vi "Keyence LJ-V7000 Read Batch Profiles(for High-Speed Mode).vi"() -> ()   [LabVIEW 2014]
doc: "This example mainly indicates how to acquire profiles in a unit of batch from controllers by using <B>Read Batch Profiles (for High-Speed Mode)</B> VI. \n\n<B>Note</B>:\nIf you execute this example, set the operation mode of the controller to the high-speed mode, and set batch measurement to ON in batch setting."
uses:
  Public/constant/Comm Interface.ctl
  Public/Clusters/Ethernet Config.ctl
  Public/Clusters/Read Batch Profile Req.ctl
  Public/constant/Batch Pos.ctl
  Public/Clusters/Read Batch Profile Rsp.ctl
  Public/Clusters/Profile Info.ctl
  State Machine State1.ctl
  Keyence LJ-V7000.lvlib
panel:
  in  "Start Monitoring":bool
  in  "Batch Stop":bool
  in  "Batch Start":bool
  out "Batch Height Image":dbl[][](graph)
  out "Profile Info":T1
  out "Profile Rsp":T2
  in  "Batch Point":u16=1000
  in  "Read Req":T3={"Read Area"=TRUE, "Batch Pos"=0, "Read Batch No"=0, "Read Profile No."=0, "Read Profile Cnt"=255, "Erase"=FALSE} {"Batch Pos" items=["CURRENT"=0, "SPECIFY"=2, "COMMITED"=3, "NEWEST PROFILE"=4]}
  in  "Stop VI":bool
  in  "Ethernet Config":T5={"IP Address"=[192, 168, 0, 1], "Port No"=24691}
  in  "Comm Interface":T6
  # "Communication Configuration"
  # "Output from Read Profiles VI"
  # "Input to Read Profiles VI"
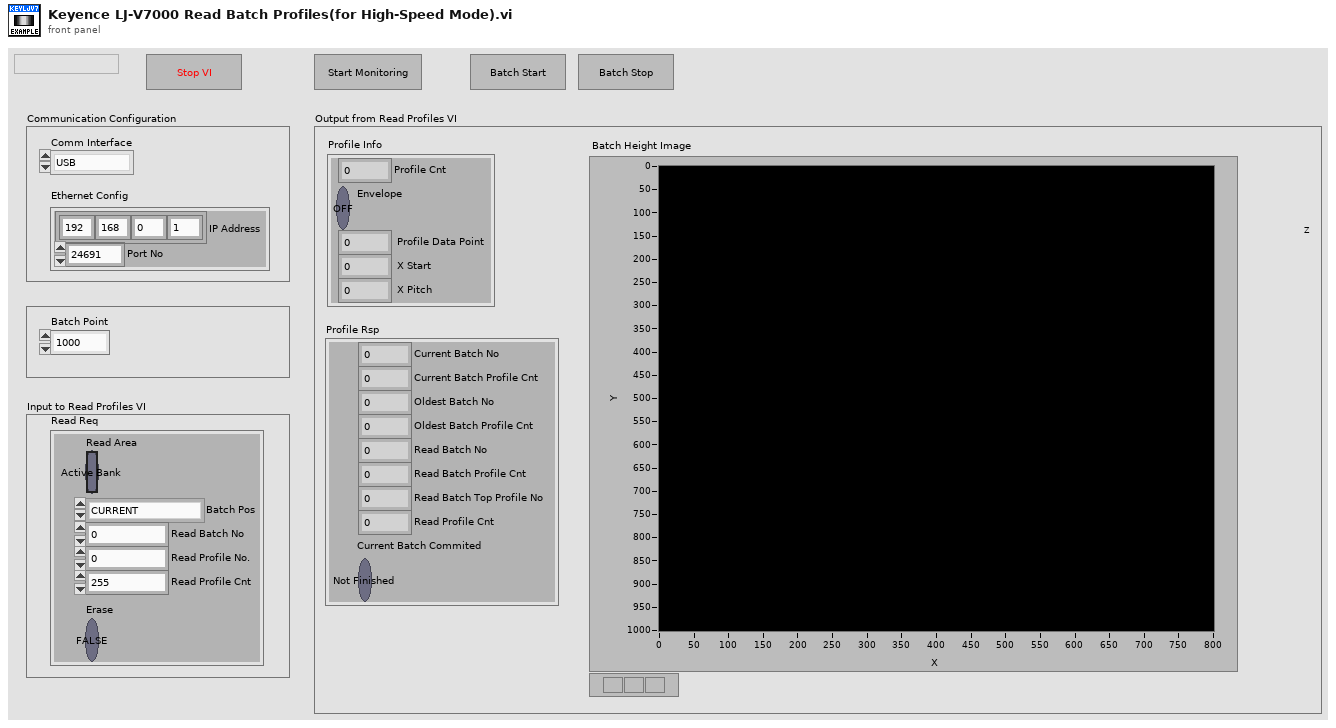
[diagram p1: front panel]
types:
  T1 = typedef "Keyence LJ-V7000.lvlib/Profile Info.ctl" = cluster{"Profile Cnt":u8, "Envelope":bool, " Profile Data Point":u16, " X Start":i32, " X Pitch":i32}
  T2 = typedef "Keyence LJ-V7000.lvlib/Read Batch Profile Rsp.ctl" = cluster{"Current Batch No":u32, "Current Batch Profile Cnt":u32, "Oldest Batch No":u32, "Oldest Batch Profile Cnt":u32, "Read Batch No":u32, "Read Batch Profile Cnt":u32, "Read Batch Top Profile No":u32, "Read Profile Cnt":u8, "Current Batch Commited":bool}
  T3 = typedef "Keyence LJ-V7000.lvlib/Read Batch Profile Req.ctl" = cluster{"Read Area":bool, "Batch Pos":T4, "Read Batch No":u32, "Read Profile No.":u32, "Read Profile Cnt":u8, "Erase":bool}
  T4 = typedef "Keyence LJ-V7000.lvlib/Batch Pos.ctl" = u8
  T5 = typedef "Keyence LJ-V7000.lvlib/Ethernet Config.ctl" = cluster{"IP Address":u8[], "Port No":u16}
  T6 = typedef "Keyence LJ-V7000.lvlib/Comm Interface.ctl" = enum8{"USB", "ETHERNET"}
  T7 = typedef "State Machine State1.ctl" = enum16{"Idle", "Batch Reading Initialize", "Batch Reading", "Batch Start", "Batch Stop", "Stop"}
  T8 = enum8{"Enabled", "Disabled", "Disabled and Grayed Out"}
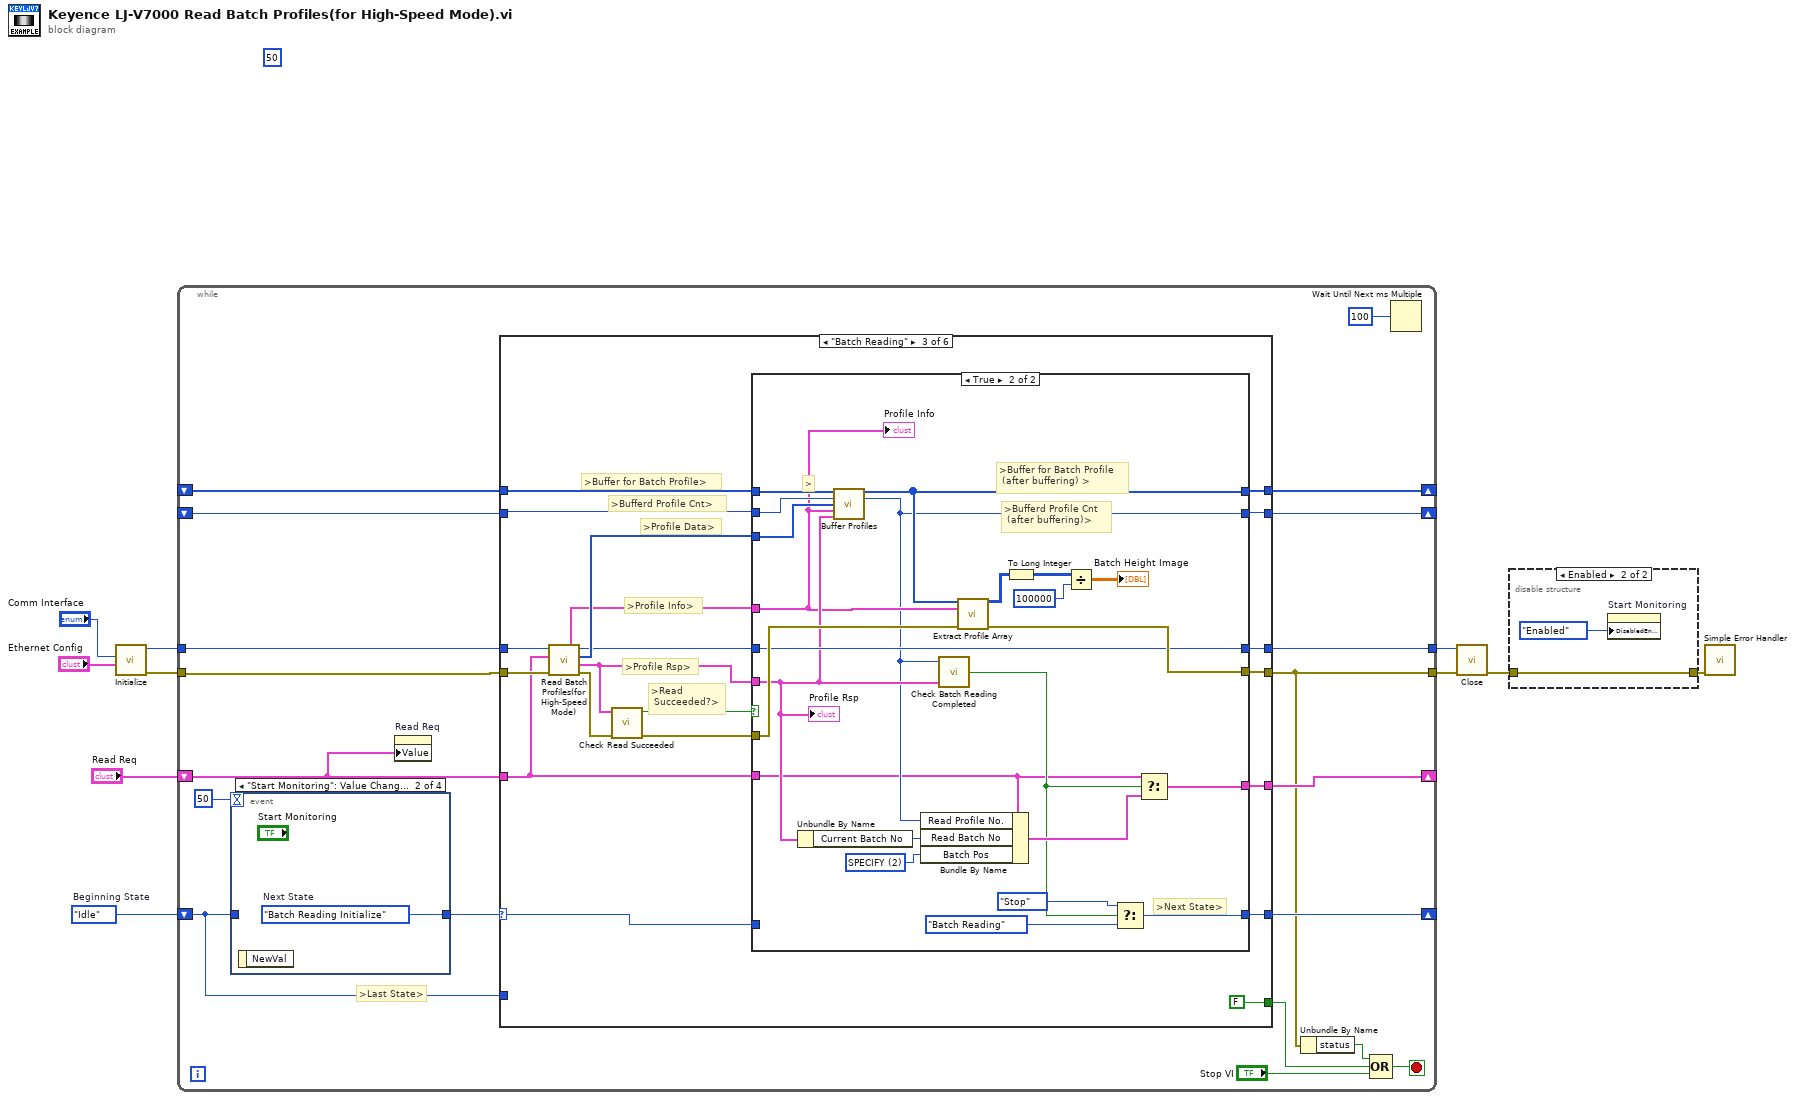
[diagram p0: block diagram]
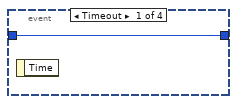
[diagram p3: hidden frame]
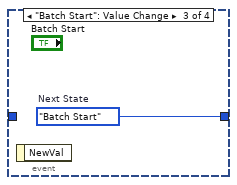
[diagram p4: hidden frame]
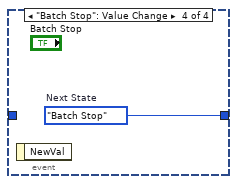
[diagram p5: hidden frame]
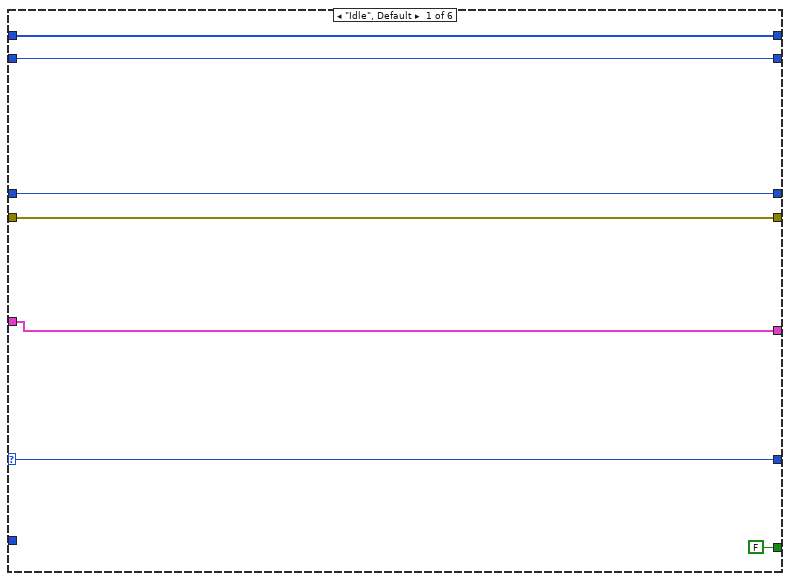
[diagram p6: hidden frame]
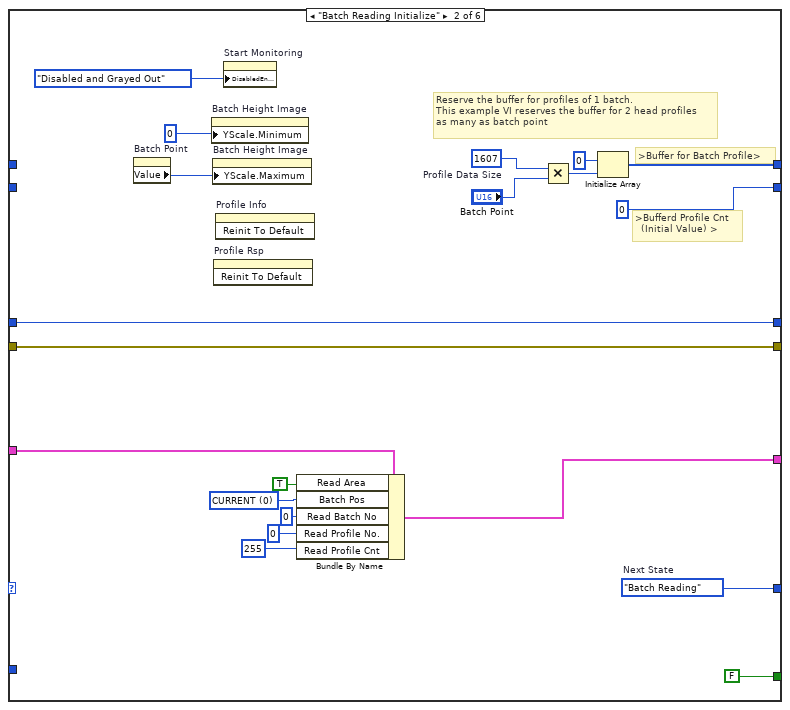
[diagram p7: hidden frame]
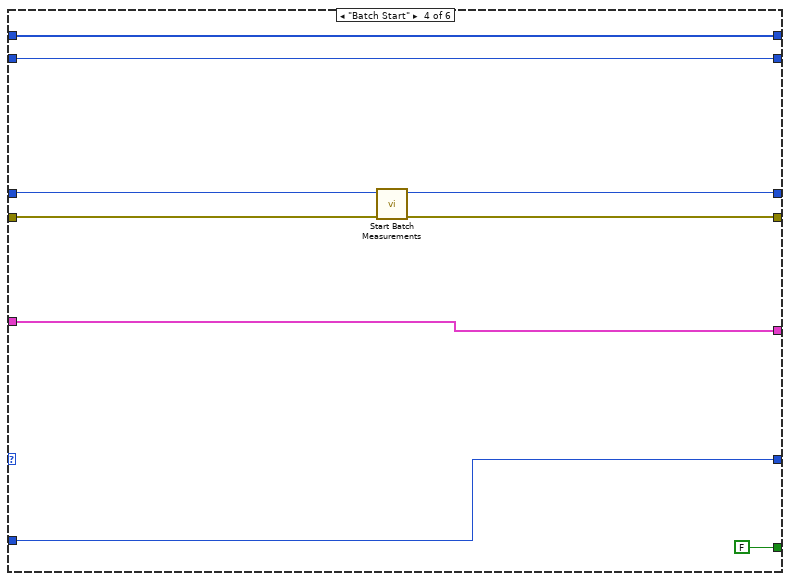
[diagram p9: hidden frame]
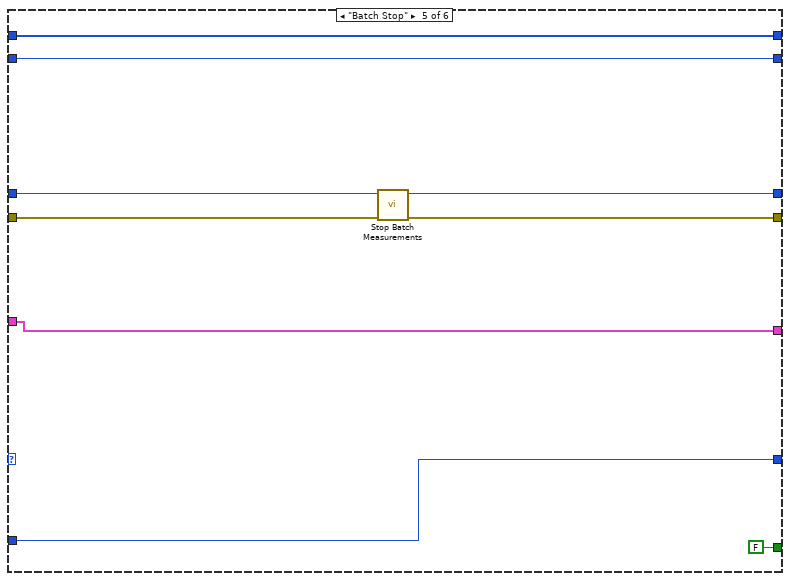
[diagram p10: hidden frame]
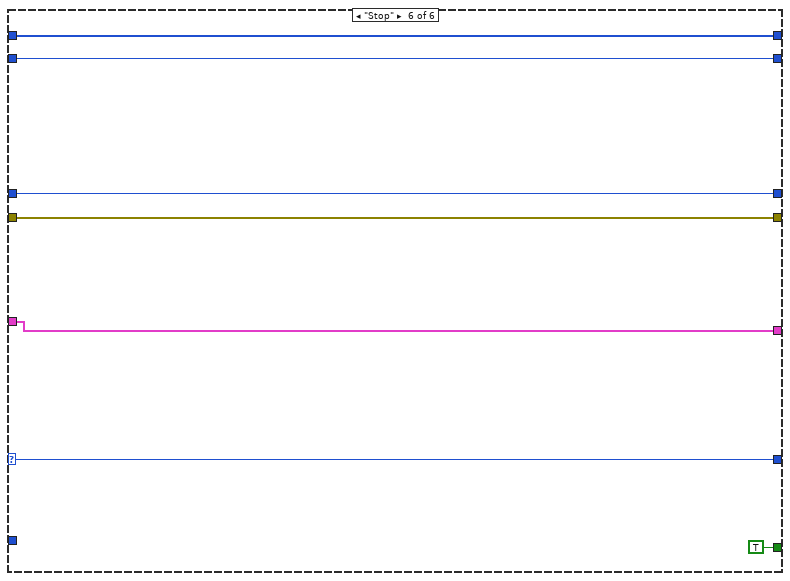
[diagram p11: hidden frame]
diagram:
  (unwired) 50
  w10 = State_Machine_State1."Idle"  # Beginning State
  n1 = call "Initialize.vi"("Ethernet Config"="Ethernet Config", "Comm Interface"="Comm Interface") -> ("error out"=w6:errorcluster, "Device ID out"=w5:i32)  [unwired: 8 in]
  n2 = while {
    shift-right: [w29] -> _
    shift-left: w10 -> [w17]
    shift-right: [w24] -> _
    shift-left: "Read Req" -> [w21]
    shift-right: [w28] -> _
    shift-left: _ -> [w26]
    shift-right: [w27] -> _
    shift-left: _ -> [w25]
    tunnel: w6 -> [w19]
    tunnel: w5 -> [w18]
    tunnel: [w13] -> w3
    tunnel: [w22] -> w4
    stop <- w12 stop-if-true
    # ">Last State>"
    n3 = event shown="[1] \"Start Monitoring\": Value Change" {
      selector: _ -> [_ _ _ _]
      dyn-events: _ -> [_ _ _ _]
      timeout: 50 -> [_ _ _ _]
      tunnel: w17 -> [w30 _ _ _]
      tunnel: [w30 w31 w32 w33] -> w20
      event Timeout {
        n4 = event-data() -> ()  [unwired: 1 in, 1 out]
      }
      event "Start Monitoring": Value Change {
        w31 = State_Machine_State1."Batch Reading Initialize"  # Next State
        n5 = event-data() -> ()  [unwired: 1 in, 1 out]
      }
      event "Batch Start": Value Change {
        w32 = State_Machine_State1."Batch Start"  # Next State
        n6 = event-data() -> ()  [unwired: 1 in, 1 out]
      }
      event "Batch Stop": Value Change {
        w33 = State_Machine_State1."Batch Stop"  # Next State
        n7 = event-data() -> ()  [unwired: 1 in, 1 out]
      }
    }
    n8 = property on="Read Req" class="Clust (strict)"("Value"=w21) -> ()  [unwired: 2 in, 2 out]
    n9 = case shown="\"Batch Reading\"" w20 {
      selector: w20 -> [w37 _ w65 _ _ w128]
      tunnel: w21 -> [w40 w60 w76 w116 w120 w134]
      tunnel: [w38 w53 w74 w118 w123 w130] -> w28
      tunnel: [w39 u32 0 w71 w117 w122 w131] -> w27
      tunnel: [w37 w51 w64 w110 w121 w128] -> w29
      tunnel: [w40 w50 w75 w116 w120 w134] -> w24
      tunnel: w18 -> [w34 w48 w80 w113 w124 w132]
      tunnel: w19 -> [w35 w49 w79 w112 w125 w133]
      tunnel: w26 -> [w38 _ w77 w118 w123 w130]
      tunnel: w25 -> [w39 _ w73 w117 w122 w131]
      tunnel: [w35 w49 w70 w111 w126 w133] -> w13
      tunnel: [w34 w48 w63 w114 w127 w132] -> w22
      tunnel: [FALSE ("Batch Reading Normally Completed") FALSE ("Batch Reading Normally Completed") FALSE ("Batch Reading Normally Completed") FALSE ("Batch Reading Normally Completed") FALSE ("Batch Reading Normally Completed") TRUE ("Batch Reading Normally Completed")] -> w14
      tunnel: w17 -> [_ _ _ w110 w121 _]
      frame "Idle", Default {
      }
      frame "Batch Reading Initialize" {
        w51 = State_Machine_State1."Batch Reading"  # Next State
        w57 = u32 1607  # Profile Data Size
        w59 = T4 0 items=["CURRENT"=0, "SPECIFY"=2, "COMMITED"=3, "NEWEST PROFILE"=4] ("Batch Pos")
        # ">Buffer for Batch Profile>"
        # ">Bufferd Profile Cnt\n  (Initial Value) >"
        # "Reserve the buffer for profiles of 1 batch.\nThis example VI reserves the buffer for 2 head profiles\nas many as batch point"
        n10 = property on="Batch Point" class="DigNum (strict)"() -> ("Value"=w42:u16)  [unwired: 2 in, 2 out]
        n11 = property on="Batch Height Image" class="IntGraph (strict)"("YScale.Minimum"=u32 0 ("Yスケール.範囲:最小値")) -> ()  [unwired: 2 in, 2 out]
        n12 = property on="Batch Height Image" class="IntGraph (strict)"("YScale.Maximum"=w42) -> ()  [unwired: 2 in, 2 out]
        n13 = invoke on="Profile Rsp" class="Clust (strict)" method="Reinit To Default"() -> ()  [unwired: 3 in, 3 out]
        n14 = invoke on="Profile Info" class="Clust (strict)" method="Reinit To Default"() -> ()  [unwired: 3 in, 3 out]
        n15 = property on="Start Monitoring" class="Bool"("DisabledEnum"=T8."Disabled and Grayed Out" ("無効")) -> ()  [unwired: 2 in, 2 out]
        n16 = Bundle By Name(cluster=w60, "Read Area"=TRUE, "Batch Pos"=w59, "Read Batch No"=u32 0, "Read Profile No."=u32 0, "Read Profile Cnt"=u8 255) -> (w50:T3)
        n17 = Multiply(x=w57, y="Batch Point") -> (x*y=w55:u32)
        n18 = Initialize Array(u32 0 ("要素"), w55) -> (w53:u32[])
      }
      frame "Batch Reading" {
        # ">Profile Data>"
        # ">Buffer for Batch Profile>"
        # ">Bufferd Profile Cnt>"
        # ">Profile Info>"
        # ">Read \n Succeeded?>"
        # ">Profile Rsp>"
        n19 = call "Read Batch Profiles(for High-Speed Mode).vi"("error in (no error)"=w79, "Read Req"=w76, "Device ID (0)"=w80) -> ("error out"=w69:errorcluster, "Profile Rsp"=w62:T2, "Profile Data"=w78:u32[], "Device ID out"=w66:i32, "Profile Info"=w72:T1)  [unwired: 4 in]
        n20 = call "Check Read Succeeded.vi"("error in (no error)"=w69, "Profile Rsp"=w62) -> ("error out"=w67:errorcluster, "Succeeded?"=w68:bool)  [unwired: 8 in]
        n21 = case shown="True" w68 {
          tunnel: w78 -> [_ w95]
          tunnel: w77 -> [w86 w96]
          tunnel: w76 -> [w84 w88]
          tunnel: [w84 w107] -> w75
          tunnel: [w86 w91] -> w74
          tunnel: w73 -> [w85 w94]
          tunnel: w72 -> [_ w92]
          tunnel: [w85 w90] -> w71
          tunnel: [w83 w103] -> w70
          tunnel: w62 -> [_ w93]
          tunnel: w67 -> [w83 w101]
          tunnel: w66 -> [w81 w98]
          tunnel: w65 -> [w82 _]
          tunnel: [w82 w99] -> w64
          tunnel: [w81 w98] -> w63
          frame False {
          }
          frame True {
            w109 = T4 2 items=["CURRENT"=0, "SPECIFY"=2, "COMMITED"=3, "NEWEST PROFILE"=4] ("Batch Pos")
            # ">Next State>"
            # ">"
            # ">Buffer for Batch Profile\n (after buffering) >"
            # ">Bufferd Profile Cnt\n (after buffering)>"
            n22 = Unbundle By Name(w93) -> ("Current Batch No"=w97:u32)
            n23 = call "Buffer Profiles.vi"("Buffer for Batch Profile\n(before buffering)"=w96, "Bufferd Profile Cnt\n(before buffering)"=w94, "Profile Data"=w95, "Profile Info"=w92, "Profile Rsp"=w93) -> (">Buffer for Batch Profile\n (after buffering) >"=w91:u32[], ">Bufferd Profile Cnt\n (after buffering)>"=w90:u32)  [unwired: 9 in]
            n24 = Bundle By Name(cluster=w88, "Read Profile No."=w90, "Read Batch No"=w97, "Batch Pos"=w109) -> (w108:T3)
            n25 = call "Check Batch Reading Completed.vi"("Profile Rsp"=w93, "Bufferd Profile Cnt"=w90) -> ("Completed?"=w89:bool)  [unwired: 3 in]
            n26 = call "Extract Profile Array.vi"("Profile Data"=w91, "Profile Info"=w92, "error in (no error)"=w101) -> ("Profile A Array1"=w105:u32[][], "error out"=w103:errorcluster)  [unwired: 8 in, 3 out]
            n27 = To Long Integer(number=w105) -> (32bit integer=w104:i32[][])
            n28 = Divide(x=w104, y=100000) -> (x/y=→"Batch Height Image":dbl[][])
            n29 = Select(t=State_Machine_State1."Stop" ("Next State"), s=w89, f=State_Machine_State1."Batch Reading" ("Next State")) -> (s? t:f=w99:T7)
            n30 = Select(t=w88, s=w89, f=w108) -> (s? t:f=w107:T3)
            "Profile Rsp" <- w93
            "Profile Info" <- w92
          }
        }
      }
      frame "Batch Start" {
        n31 = call "Start Batch Measurements.vi"("error in (no error)"=w112, "Device ID (0)"=w113) -> ("error out"=w111:errorcluster, "Device ID out"=w114:i32)  [unwired: 8 in]
      }
      frame "Batch Stop" {
        n32 = call "Stop Batch Measurements.vi"("error in (no error)"=w125, "Device ID (0)"=w124) -> ("error out"=w126:errorcluster, "Device ID out"=w127:i32)  [unwired: 8 in]
      }
      frame "Stop" {
      }
    }
    n33 = Unbundle By Name(w13) -> ("status"=w11:bool)
    n34 = Compound Arithmetic op=OR(w11, w14, "Stop VI") -> (w12:bool)
    n35 = Wait Until Next ms Multiple(millisecond multiple=u32 100 ("ミリ秒倍数")) -> ()  [unwired: 1 out]
  }
  n36 = call "Close.vi"("error in (no error)"=w3, "Device ID (0)"=w4) -> ("error out"=w1:errorcluster)  [unwired: 8 in, 1 out]
  n37 = disable-structure shown="Enabled" {
    disable-tunnel: w1 -> [w135 w137]
    disable-tunnel: [w135 w137] -> w2
    frame Disabled {
    }
    frame Enabled {
      n38 = property on="Start Monitoring" class="Bool"("DisabledEnum"=T8."Enabled" ("無効")) -> ()  [unwired: 2 in, 2 out]
    }
  }
  n39 = call <vilib>:"Simple Error Handler.vi"("error in (no error)"=w2) -> ()  [unwired: 4 in, 5 out]
